vi "Delay.vi"(8 "error in (no error)":errorcluster, 10 "Delay Time (10 ms)":i32=10, 11 "VISA resource name":refnum<visa-resource-name>) -> (0 "error out":errorcluster, 3 "VISA resource name out":refnum<visa-resource-name>)   [LabVIEW 2024, in "BK Precision 8500B Series.lvlib"]
doc: "Creates a time delay in milliseconds."
uses:
  BK Precision 8500B Series.lvlib
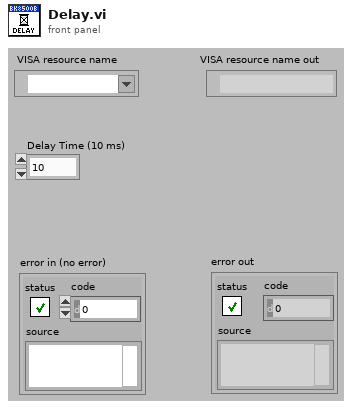
[diagram p1: front panel]
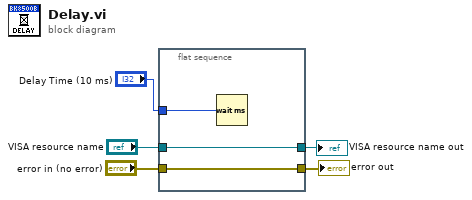
[diagram p0: block diagram]
diagram:
  n1 = flat-sequence {
    tunnel: "Delay Time (10 ms)" -> [w8]
    tunnel: [w7] -> w4
    tunnel: "VISA resource name" -> [w7]
    tunnel: [w6] -> w2
    tunnel: "error in (no error)" -> [w6]
    frame #0 {
      n2 = Wait (ms)(milliseconds to wait=w8) -> ()  [unwired: 1 out]
    }
  }
  "error out" <- w2
  "VISA resource name out" <- w4
